vi "Find FRF Info from File Lines.vi"(5 "error in (no error)":errorcluster, 7 "Line text":string[](array[string])) -> (13 "Channel Lines info":T1(array[cluster]), 19 "error out":errorcluster)   [LabVIEW 2022 SP3, in "Nastran PCH.lvclass"]
uses:
  Nastran PCH.lvclass
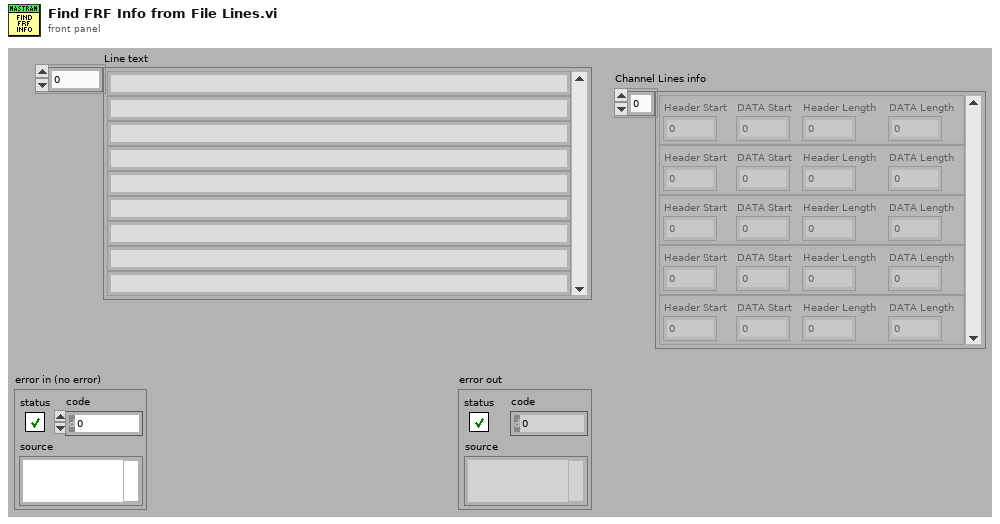
[diagram p1: front panel]
types:
  T1 = cluster{"Header Start":i32, "DATA Start":i32, "Header Length":i32, "DATA Length":i32}[]
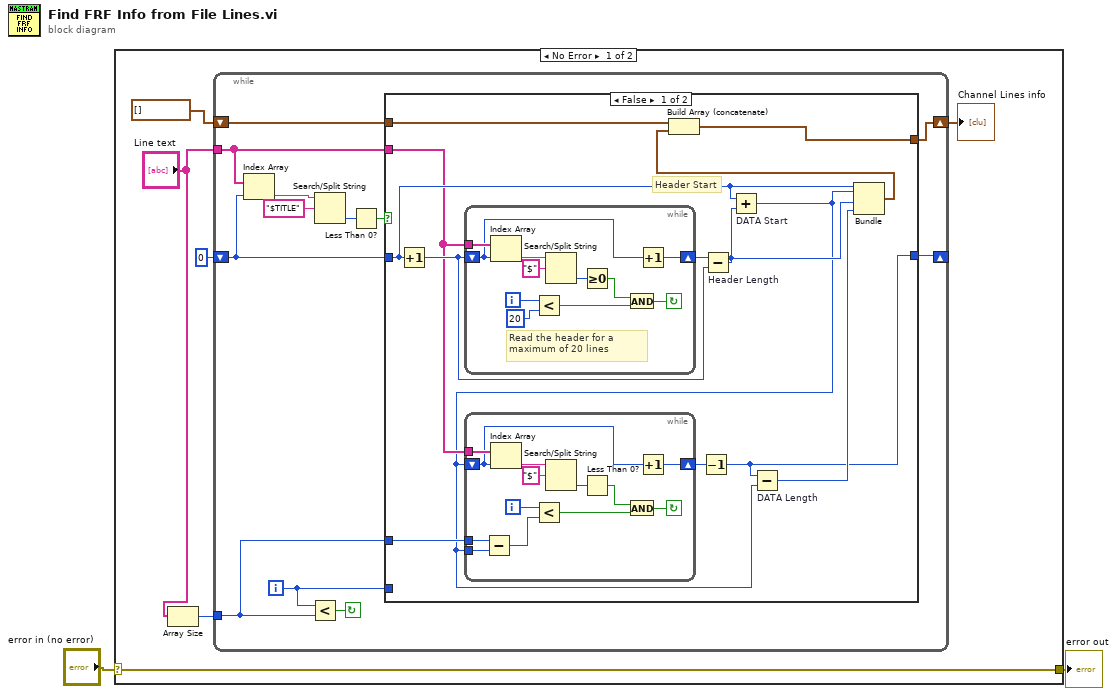
[diagram p0: block diagram]
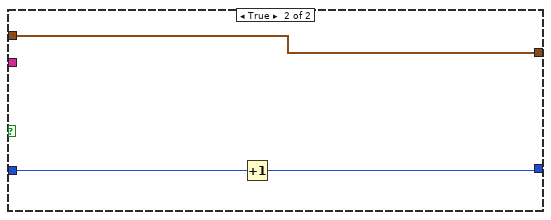
[diagram p2: hidden frame]
diagram:
  n1 = case shown="No Error" "error in (no error)" {
    selector: "error in (no error)" -> [w8 w61]
    tunnel: [w8 w61] -> w1
    frame No Error {
      n2 = Array Size(array="Line text") -> (size(s)=w5:i32)
      n3 = while {
        tunnel: "Line text" -> [w11]
        shift-right: [w17] -> w3
        shift-left: cluster{i32, i32, i32, i32}[] [] -> [w16]
        shift-right: [w9] -> _
        shift-left: 0 -> [w12]
        tunnel: w5 -> [w10]
        i -> [w15]
        stop <- w14 continue-if-true
        n4 = Index Array(array=w11, index=w12) -> (element=w13:string)
        n5 = Less?(x=w15, y=w10) -> (x < y?=w14:bool)
        n6 = Search/Split String(string=w13, search string/char (-)="$TITLE") -> (offset of match=w19:i32)  [unwired: 3 out]
        n7 = Less Than 0?(x=w19) -> (x < 0?=w18:bool)
        n8 = case shown="False" w18 {
          tunnel: w15 -> [_ _]
          tunnel: [w33 w60] -> w17
          tunnel: w16 -> [w32 w60]
          tunnel: w12 -> [w28 w59]
          tunnel: w11 -> [w27 _]
          tunnel: w10 -> [w26 _]
          tunnel: [w21 w58] -> w9
          frame False {
            # "Header Start"
            n9 = Increment(x=w28) -> (x+1=w30:i32)
            n10 = while {
              shift-right: [w48] -> w31
              shift-left: w30 -> [w47]
              tunnel: w27 -> [w54]
              i -> [w55]
              stop <- w49 continue-if-true
              # "Read the header for a maximum of 20 lines"
              n11 = Index Array(array=w54, index=w47) -> (element=w53:string)
              n12 = Less?(x=w55, y=20) -> (x < y?=w50:bool)
              n13 = Search/Split String(string=w53, search string/char (-)="$") -> (offset of match=w56:i32)  [unwired: 3 out]
              n14 = Greater Or Equal To 0?(x=w56) -> (x >= 0?=w51:bool)
              n15 = And(x=w51, y=w50) -> (x .and. y?=w49:bool)
              n16 = Increment(x=w47) -> (x+1=w48:i32)
            }
            n17 = Subtract "Header Length"(x=w31, y=w30) -> (x-y=w29:i32)
            n18 = Add "DATA Start"(x=w28, y=w29) -> (x+y=w24:i32)
            n19 = while {
              shift-right: [w38] -> w23
              shift-left: w24 -> [w37]
              tunnel: w27 -> [w44]
              tunnel: w26 -> [w36]
              tunnel: w24 -> [w35]
              i -> [w45]
              stop <- w39 continue-if-true
              n20 = Subtract(x=w36, y=w35) -> (x-y=w34:i32)
              n21 = Index Array(array=w44, index=w37) -> (element=w43:string)
              n22 = Less?(x=w45, y=w34) -> (x < y?=w40:bool)
              n23 = Search/Split String(string=w43, search string/char (-)="$") -> (offset of match=w46:i32)  [unwired: 3 out]
              n24 = Less Than 0?(x=w46) -> (x < 0?=w41:bool)
              n25 = And(x=w41, y=w40) -> (x .and. y?=w39:bool)
              n26 = Increment(x=w37) -> (x+1=w38:i32)
            }
            n27 = Decrement(x=w23) -> (x-1=w21:i32)
            n28 = Subtract "DATA Length"(x=w21, y=w24) -> (x-y=w22:i32)
            n29 = Bundle(w28, w24, w29, w22) -> (w25:cluster{i32, i32, i32, i32})  [unwired: 1 out]
            n30 = Build Array (concatenate)(w32, w25) -> (w33:cluster{i32, i32, i32, i32}[])
          }
          frame True {
            n31 = Increment(x=w59) -> (x+1=w58:i32)
          }
        }
      }
      "Channel Lines info" <- w3
    }
    frame Error {
    }
  }
  "error out" <- w1
